vi "MenuOptions.vi"(8 "error in":errorcluster, 9 "VI ref":refnum<vi>, 11 "menu ref in":refnum<k9>) -> (0 "error out":errorcluster, 3 "menu ref out":refnum<k9>)   [LabVIEW 2014, in "SPI Configuration Tool.lvlib"]
doc: "This VI configures the application menu options. If you need aditional menu items add them in this VI."
uses:
  SPI Configuration Tool.lvlib
  <vilib>/Utility/miscctls.llb/LVMenuShortCut.ctl
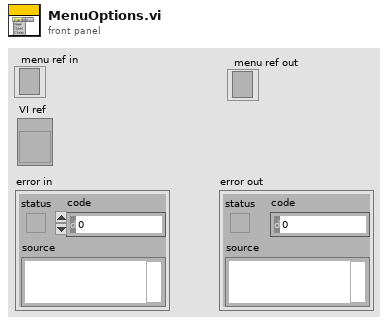
[diagram p1: front panel]
types:
  T1 = typedef "LVMenuShortCut.ctl" = cluster{"Include Shift Key?":bool, "Include Ctrl Key?":bool, "Shortcut Key":string}
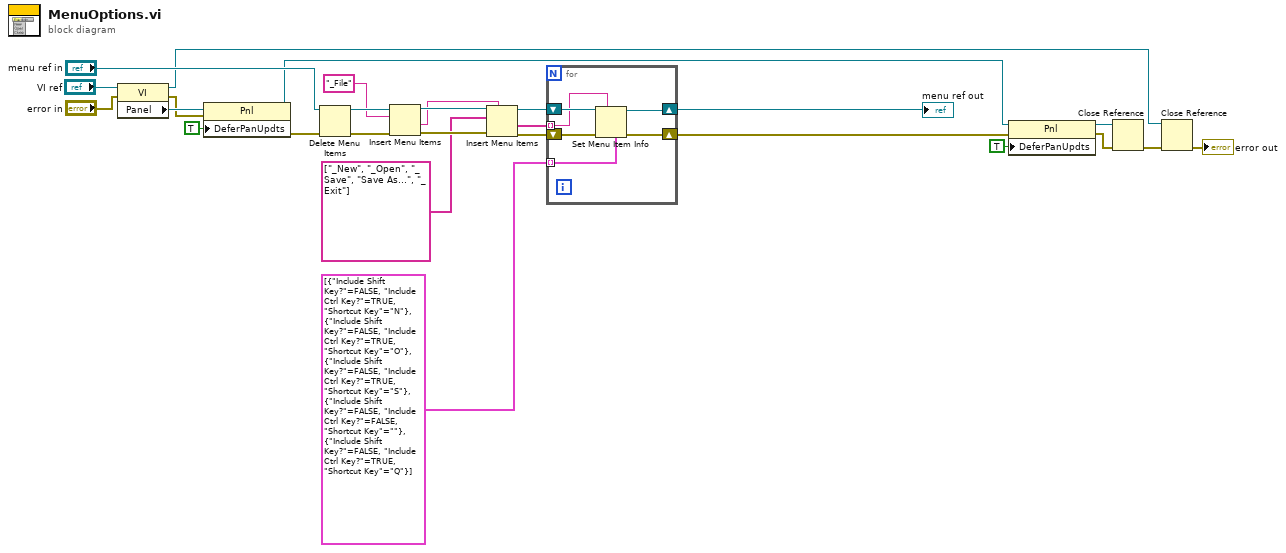
[diagram p0: block diagram]
diagram:
  n1 = property class="VI"(reference="VI ref", error in="error in") -> (reference out=w12:refnum<vi>, error out=w8:errorcluster, "Panel"=w11:refnum<vi>)
  n2 = property class="Pnl"(reference=w11, error in=w8, "DeferPanUpdts"=TRUE ("Defer Panel Updates")) -> (reference out=w5:refnum<vi>, error out=w7:errorcluster)
  n3 = Delete Menu Items(6:w7, 9:"menu ref in") -> (0:w22:errorcluster, 3:w26:refnum<k9>)  [unwired: 2 in]
  n4 = Insert Menu Items(6:w22, 8:"_File", 9:w26) -> (0:w21:errorcluster, 1:w23:string, 3:w24:refnum<k9>)  [unwired: 3 in]
  n5 = Insert Menu Items(5:w23, 6:w21, 8:string[] ["_New", "_Open", "_Save", "Save As...", "_Exit"] ("item names"), 9:w24) -> (0:w18:errorcluster, 1:w17:string[], 3:w19:refnum<k9>)  [unwired: 2 in]
  n6 = for {
    shift-right: [w31] -> w15
    shift-left: w19 -> [w33]
    tunnel: w17 -> [w30] mode=indexing
    tunnel: T1[] [{"Include Shift Key?"=FALSE, "Include Ctrl Key?"=TRUE, "Shortcut Key"="N"}, {"Include Shift Key?"=FALSE, "Include Ctrl Key?"=TRUE, "Shortcut Key"="O"}, {"Include Shift Key?"=FALSE, "Include Ctrl Key?"=TRUE, "Shortcut Key"="S"}, {"Include Shift Key?"=FALSE, "Include Ctrl Key?"=FALSE, "Shortcut Key"=""}, {"Include Shift Key?"=FALSE, "Include Ctrl Key?"=TRUE, "Shortcut Key"="Q"}] -> [w28] mode=indexing
    shift-right: [w29] -> w14
    shift-left: w18 -> [w32]
    n7 = Set Menu Item Info(4:w28, 7:w30, 8:w32, 11:w33) -> (0:w29:errorcluster, 3:w31:refnum<k9>)  [unwired: 3 in]
  }
  "menu ref out" <- w15
  n8 = property class="Pnl"(reference=w5, error in=w14, "DeferPanUpdts"=TRUE ("Defer Panel Updates")) -> (reference out=w4:refnum<vi>, error out=w3:errorcluster)
  n9 = Close Reference(reference=w4, error in (no error)=w3) -> (error out=w2:errorcluster)
  n10 = Close Reference(reference=w12, error in (no error)=w2) -> (error out=→"error out":errorcluster)
